vi "2 RIO.vi"(8 "Error In":errorcluster, 9 "Manual Override Cluster":T1, 10 "Sensor Data":T5 {"Robot Heading" format="%05.1f"; "Wind Direction" format="%05.1f"}, 11 "MissionQueue In":refnum<class "MissionQueue.lvclass">) -> (0 "Error Out":errorcluster, 2 "Setpoints to Boat":T2, 3 "MissionQueue Out":refnum<class "MissionQueue.lvclass">)   [LabVIEW 2011]
uses:
  2 Typedefs/sensorData.ctl
  2 Typedefs/UTM Location.ctl
  2 Typedefs/heading.ctl
  Classes/Missions/MissionQueue/MissionQueue.lvclass
  2 Typedefs/setpoints to boat.ctl
  2 Typedefs/sail setpt.ctl
  2 Typedefs/rudder angle.ctl
  2 Typedefs/manual override.ctl
  2 Globals/2 Global.vi
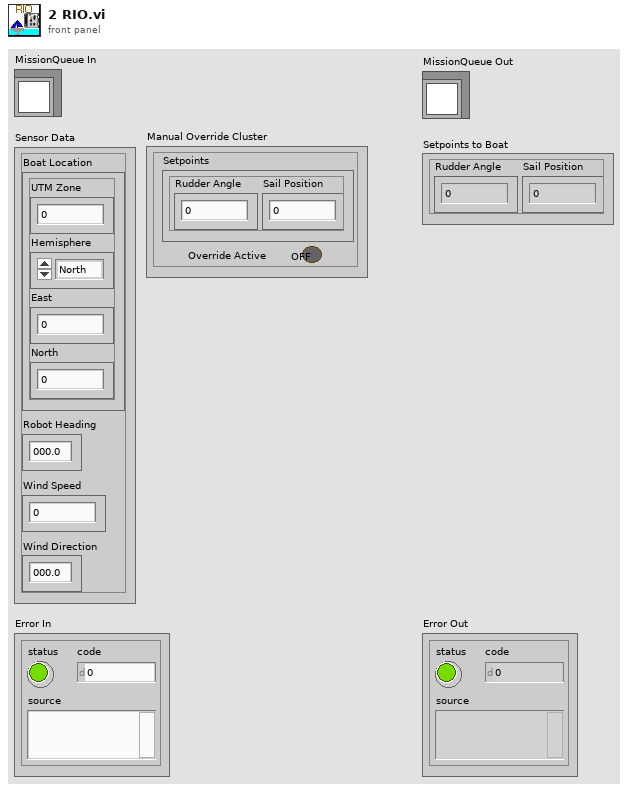
[diagram p1: front panel]
types:
  T1 = typedef "manual override.ctl" = cluster{"Override Active":bool, "Setpoints":T2}
  T2 = typedef "setpoints to boat.ctl" = cluster{"Sail Position":T3, "Rudder Angle":T4}
  T3 = typedef "sail setpt.ctl" = dbl
  T4 = typedef "rudder angle.ctl" = dbl
  T5 = typedef "sensorData.ctl" = cluster{"Boat Location":T6, "Robot Heading ":T7, "Wind Speed":dbl, "Wind Direction":T7}
  T6 = typedef "UTM Location.ctl" = cluster{"UTM Zone":dbl, "Hemisphere":enum16{"North", "South"}, "East":dbl, "North":dbl}
  T7 = typedef "heading.ctl" = dbl
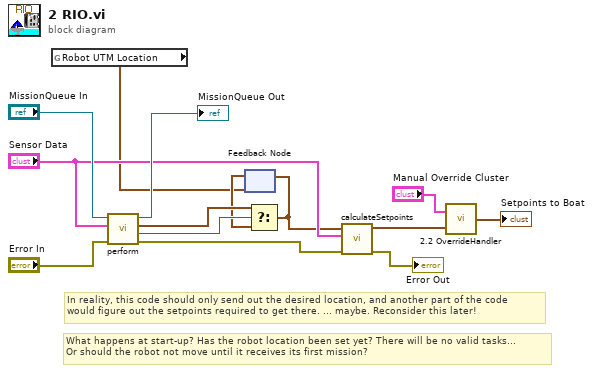
[diagram p0: block diagram]
diagram:
  # "What happens at start-up? Has the robot location been set yet? There will be no valid tasks...\nOr should the robot not move until it receives its first mission?"
  # "In reality, this code should only send out the desired location, and another part of the code\nwould figure out the setpoints required to get there. ... maybe. Reconsider this later!"
  n1 = global read "2 Global.vi" "Robot UTM Location"() -> (w1:T6)
  n2 = call "perform.vi"("error in (no error)"="Error In", "Sensor Data"="Sensor Data", "MissionQueue in"="MissionQueue In") -> ("error out"=w8:errorcluster, "Valid?"=w5:bool, "Desired Location"=w4:T6, "MissionQueue out"=→"MissionQueue Out":refnum<class "MissionQueue.lvclass">)  [unwired: 5 in]
  n3 = feedback #1(w1) -> (w2:T6)
  n4 = Select(t=w4, s=w5, f=w2) -> (s? t:f=w3:T6)
  n5 = feedback-in #1(w3) -> ()
  n6 = call "calculateSetpoints.vi"("error in (no error)"=w8, "Sensor Data"="Sensor Data", "Desired Location"=w3) -> ("error out"=→"Error Out":errorcluster, "Setpoints"=w14:T2)  [unwired: 7 in]
  n7 = call "2.2 OverrideHandler.vi"("Think Setpoints"=w14, "Manual Override Cluster"="Manual Override Cluster") -> ("Setpoints to Boat"=→"Setpoints to Boat":T2)
